vi "test harness_FXP_Linear_controller_observer.vi"(8 "error in (no error)":errorcluster, 11 "TestCase in":refnum<class "FXP_observer_TestCase.lvclass">) -> (0 "error out":errorcluster, 3 "TestCase out":refnum<class "FXP_observer_TestCase.lvclass">)   [LabVIEW 2017, in "FXP_observer_TestCase.lvclass"]
uses:
  FXP_observer_TestCase.lvclass
  <vilib>/rvi/DesktopExecutionNode/Execution/niFpgaDEN_Execute.vi
  <vilib>/rvi/DesktopExecutionNode/DesktopExecutionNode.xnode
panel:
  out "output array":fxp<+/-,51,11>[](array[numeric])
  out "xk_1_2":fxp<+/-,32,8>[](array[numeric])
  out "xerr":fxp<+/-,32,5>[](array[numeric])
  out "error A*x_k_1":errorcluster
  out "Numeric":dbl
  out "del u(k)":fxp<+/-,64,15>
  out "u_k (saturated)":fxp<+/-,32,5>
  out "A*x 2":fxp<+/-,32,7>[](array[numeric])
  out "error (xk_1_1)":errorcluster
  out "error (ydest)":errorcluster
  out "x+y":fxp<+/-,51,11>[](array[numeric])
  out "Az_mat in":fxp<+/-,32,5>[][](array[numeric])
  in  "du_umax":fxp<+/-,18,5>
  in  "xk_1_0":fxp<+/-,32,5>[](array[numeric])=[0.0, 0.0, 0.0, 0.0, 0.0, 0.0, 0.0, 0.0, 0.0, 0.0, 0.0, 0.0, 0.0, 0.0, 0.0, 0.0, 0.0, 0.0, 0.0, 0.0, 0.0, 0.0, 0.0, 0.0, 0.0, 0.0, 0.0, 0.0, 0.0, 0.0, 0.0, 0.0, 0.0, 0.0, 0.0, 0.0, 0.0, 0.0, 0.0, 0.0, 0.0, 0.0, 0.0, 0.0, 0.0, 0.0, 0.0, 0.0, 0.0, 0.0]
  in  "x_u(k)":fxp<+/-,32,8>
  in  "ControlParams_distEst":T1={"umax"=0.0, "NS"=0, "ref_f_VEC"=[0.0, 0.0], "Nu11_22"=[0.0, 0.0], "u0"=[0.0, 0.0]}
  in  "u(k-1)":fxp<+/-,18,5>=0.14501953125
  in  "y(k)":fxp<+/-,18,5>=0.123046875
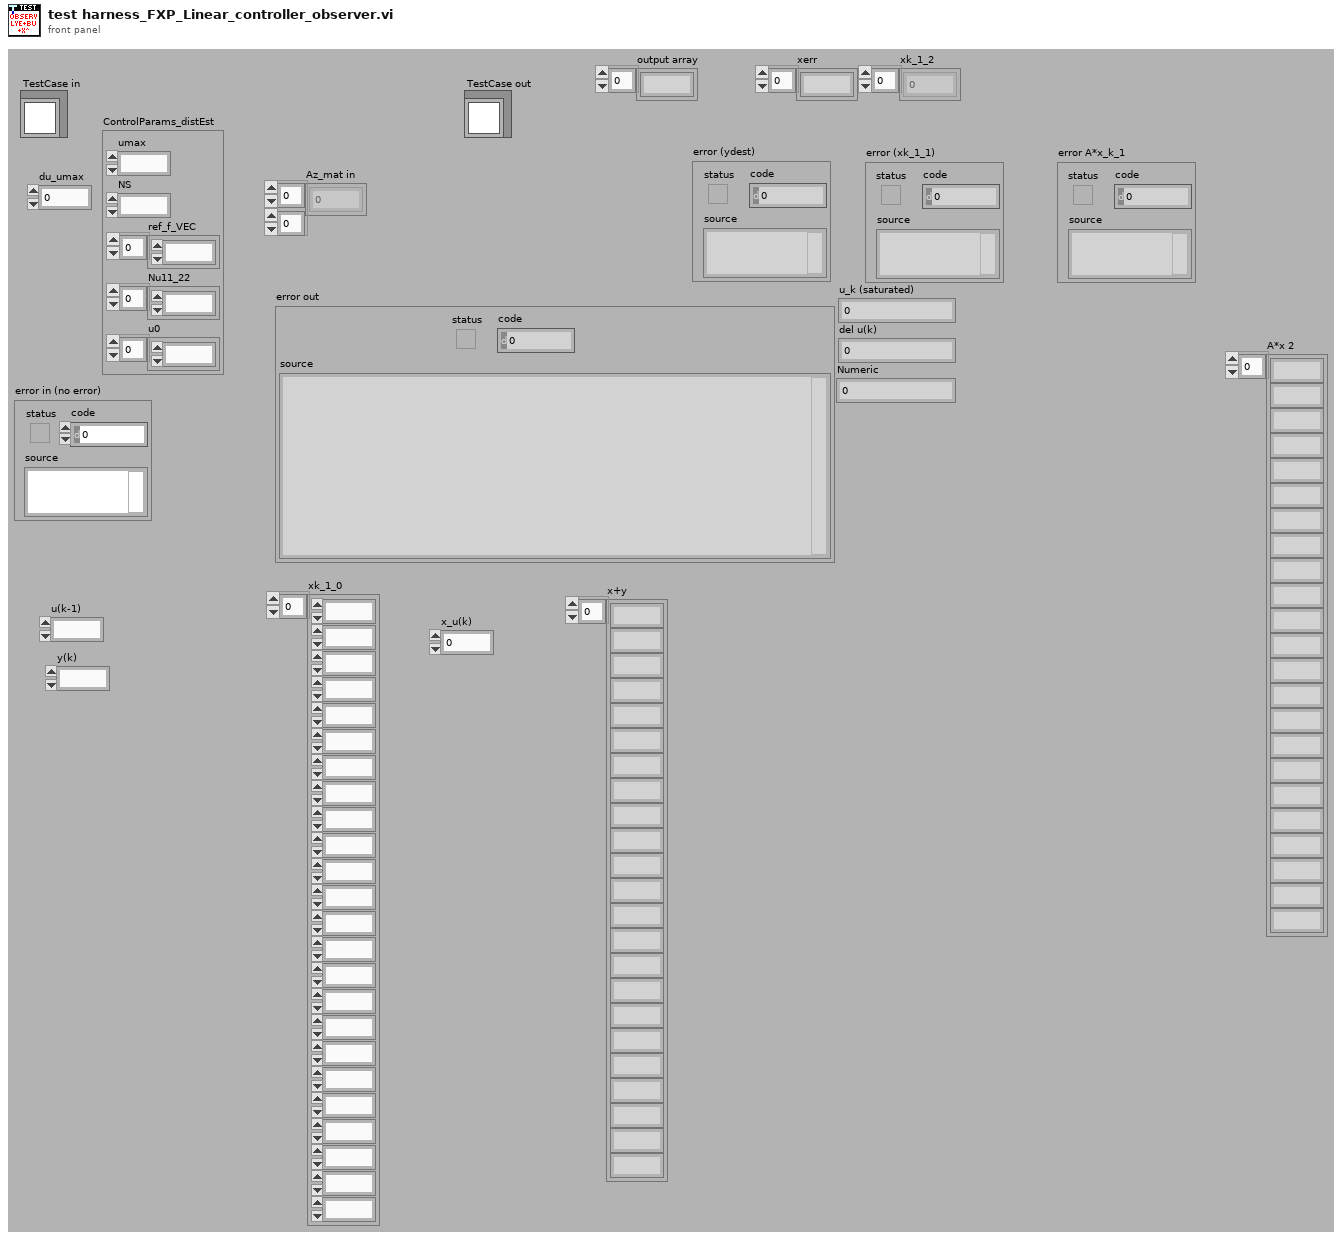
[diagram p1: front panel]
types:
  T1 = cluster{"umax":fxp<+/-,18,5>, "NS":u8, "ref_f_VEC":fxp<+/-,32,5>[], "Nu11_22":fxp<+/-,32,5>[], "u0":fxp<+/-,32,5>[]}
  T2 = cluster{"Bz":fxp<+/-,32,5>[], "Ldist":fxp<+/-,32,5>[], "Kz":fxp<+/-,32,15>[], "Nx":fxp<+/-,32,5>[], "Ax_col":fxp<+/-,32,5>[]}
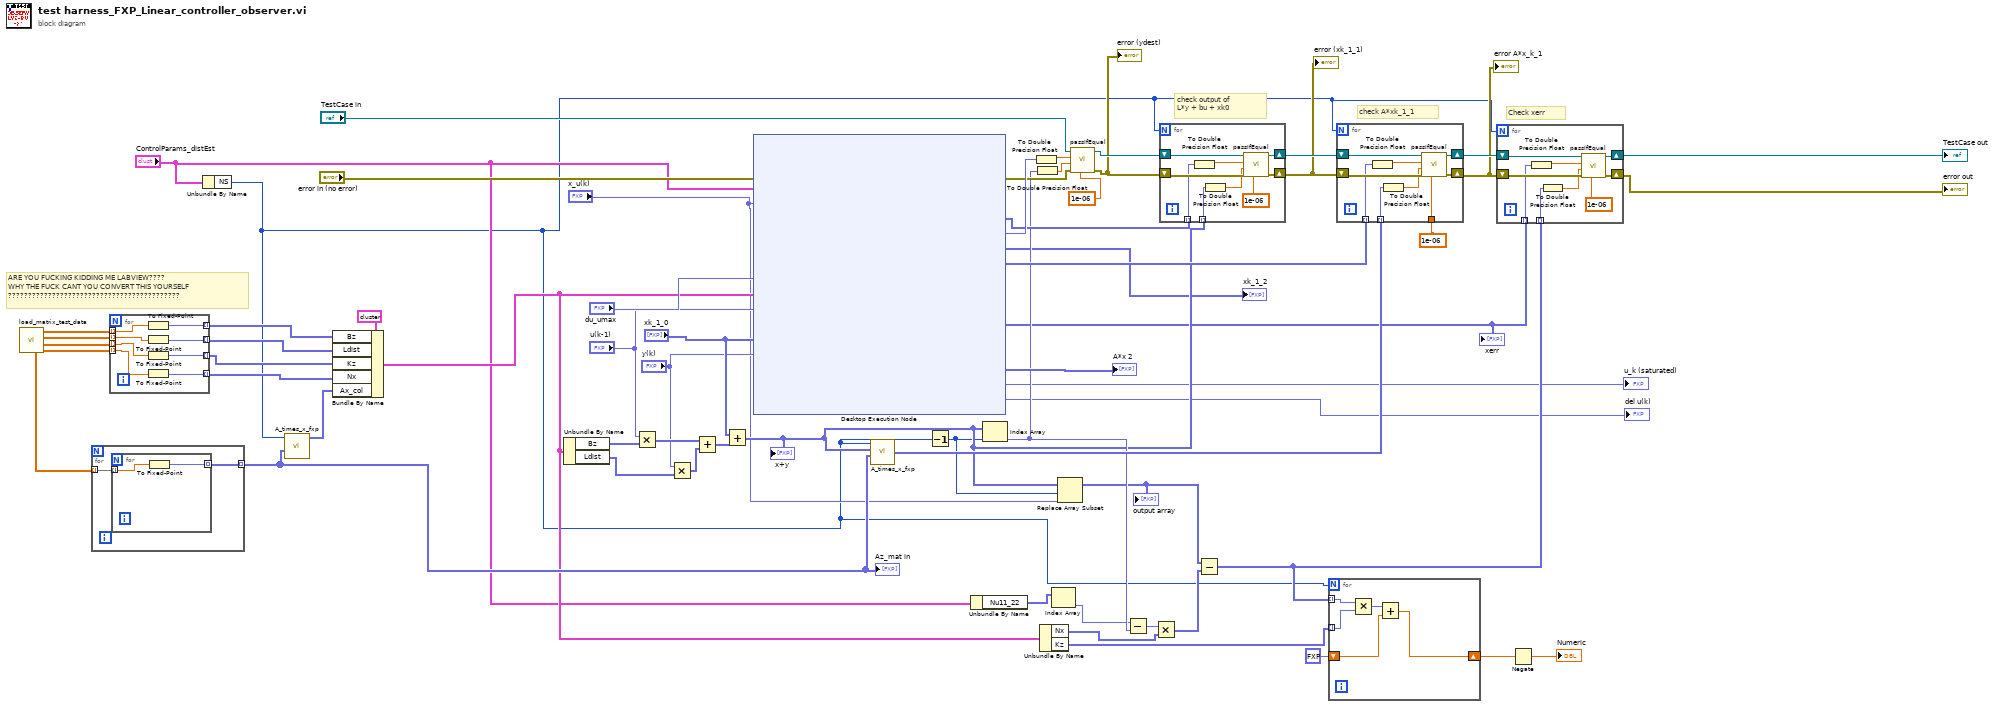
[diagram p0: block diagram]
diagram:
  # "check A*xk_1_1"
  # "check output of \nL*y + bu + xk0"
  # "Check xerr"
  # "ARE YOU FUCKING KIDDING ME LABVIEW????\nWHY THE FUCK CANT YOU CONVERT THIS YOURSELF\n???????????????????????????????????????????"
  n1 = call "load_matrix_test_data.vi"() -> ("Nx"=w57:dbl[], "Kz"=w58:dbl[], "Lz"=w59:dbl[], "Bz"=w60:dbl[], "A_mat"=w56:dbl[][])  [unwired: 5 in, 2 out]
  n2 = for {
    tunnel: [w65] -> w43 mode=indexing
    tunnel: w56 -> [w64] mode=indexing
    n3 = for {
      tunnel: w64 -> [w67] mode=indexing
      tunnel: [w66] -> w65 mode=indexing
      n4 = To Fixed-Point(number=w67) -> (fixed-point=w66:fxp<+/-,32,5>)  [unwired: 1 in]
    }
  }
  "Az_mat in" <- w43
  n5 = for {
    tunnel: w60 -> [w75] mode=indexing
    tunnel: w59 -> [w74] mode=indexing
    tunnel: w58 -> [w73] mode=indexing
    tunnel: w57 -> [w72] mode=indexing
    tunnel: [w71] -> w54 mode=indexing
    tunnel: [w70] -> w53 mode=indexing
    tunnel: [w69] -> w3 mode=indexing
    tunnel: [w68] -> w52 mode=indexing
    n6 = To Fixed-Point(number=w75) -> (fixed-point=w71:fxp<+/-,32,5>)  [unwired: 1 in]
    n7 = To Fixed-Point(number=w74) -> (fixed-point=w70:fxp<+/-,32,5>)  [unwired: 1 in]
    n8 = To Fixed-Point(number=w73) -> (fixed-point=w69:fxp<+/-,32,15>)  [unwired: 1 in]
    n9 = To Fixed-Point(number=w72) -> (fixed-point=w68:fxp<+/-,32,5>)  [unwired: 1 in]
  }
  n10 = Unbundle By Name("ControlParams_distEst") -> ("NS"=w1:u8)
  n11 = call "A_times_x_fxp.vi"("Az_mat in"=w43, "NS"=w1) -> ("Az_vec out"=w51:fxp<+/-,32,5>[])  [unwired: 8 in, 1 out]
  n12 = Bundle By Name(cluster=T2 {"Bz"=[0.0, 0.0, 0.0, 0.0, 0.0, 0.0, 0.0, 0.0, 0.0, 0.0, 0.0, 0.0, 0.0, 0.0, 0.0, 0.0, 0.0, 0.0, 0.0, 0.0, 0.0, 0.0, 0.0, 0.0, 0.0, 0.0, 0.0, 0.0, 0.0, 0.0, 0.0, 0.0, 0.0, 0.0, 0.0, 0.0, 0.0, 0.0, 0.0, 0.0, 0.0, 0.0, 0.0, 0.0, 0.0, 0.0, 0.0, 0.0, 0.0, 0.0], "Ldist"=[0.0, 0.0, 0.0, 0.0, 0.0, 0.0, 0.0, 0.0, 0.0, 0.0, 0.0, 0.0, 0.0, 0.0, 0.0, 0.0, 0.0, 0.0, 0.0, 0.0, 0.0, 0.0, 0.0, 0.0, 0.0, 0.0, 0.0, 0.0, 0.0, 0.0, 0.0, 0.0, 0.0, 0.0, 0.0, 0.0, 0.0, 0.0, 0.0, 0.0, 0.0, 0.0, 0.0, 0.0, 0.0, 0.0, 0.0, 0.0, 0.0, 0.0], "Kz"=[0.0, 0.0, 0.0, 0.0, 0.0, 0.0, 0.0, 0.0, 0.0, 0.0, 0.0, 0.0, 0.0, 0.0, 0.0, 0.0, 0.0, 0.0, 0.0, 0.0, 0.0, 0.0, 0.0, 0.0, 0.0, 0.0, 0.0, 0.0, 0.0, 0.0, 0.0, 0.0, 0.0, 0.0, 0.0, 0.0, 0.0, 0.0, 0.0, 0.0, 0.0, 0.0, 0.0, 0.0, 0.0, 0.0, 0.0, 0.0, 0.0, 0.0], "Nx"=[0.0, 0.0, 0.0, 0.0, 0.0, 0.0, 0.0, 0.0, 0.0, 0.0, 0.0, 0.0, 0.0, 0.0, 0.0, 0.0, 0.0, 0.0, 0.0, 0.0, 0.0, 0.0, 0.0, 0.0, 0.0, 0.0, 0.0, 0.0, 0.0, 0.0, 0.0, 0.0, 0.0, 0.0, 0.0, 0.0, 0.0, 0.0, 0.0, 0.0, 0.0, 0.0, 0.0, 0.0, 0.0, 0.0, 0.0, 0.0, 0.0, 0.0], "Ax_col"=[0.0, 0.0, 0.0, 0.0, 0.0, 0.0, 0.0, 0.0, 0.0, 0.0, 0.0, 0.0, 0.0, 0.0, 0.0, 0.0, 0.0, 0.0, 0.0, 0.0, 0.0, 0.0, 0.0, 0.0, 0.0, 0.0, 0.0, 0.0, 0.0, 0.0, 0.0, 0.0, 0.0, 0.0, 0.0, 0.0, 0.0, 0.0, 0.0, 0.0, 0.0, 0.0, 0.0, 0.0, 0.0, 0.0, 0.0, 0.0, 0.0, 0.0, 0.0, 0.0, 0.0, 0.0, 0.0, 0.0, 0.0, 0.0, 0.0, 0.0, 0.0, 0.0, 0.0, 0.0, 0.0, 0.0, 0.0, 0.0, 0.0, 0.0, 0.0, 0.0, 0.0, 0.0, 0.0, 0.0, 0.0, 0.0, 0.0, 0.0, 0.0, 0.0, 0.0, 0.0, 0.0, 0.0, 0.0, 0.0, 0.0, 0.0, 0.0, 0.0, 0.0, 0.0, 0.0, 0.0, 0.0, 0.0, 0.0, 0.0, 0.0, 0.0, 0.0, 0.0, 0.0, 0.0, 0.0, 0.0, 0.0, 0.0, 0.0, 0.0, 0.0, 0.0, 0.0, 0.0, 0.0, 0.0, 0.0, 0.0, 0.0, 0.0, 0.0, 0.0, 0.0, 0.0, 0.0, 0.0, 0.0, 0.0, 0.0, 0.0, 0.0, 0.0, 0.0, 0.0, 0.0, 0.0, 0.0, 0.0, 0.0, 0.0, 0.0, 0.0, 0.0, 0.0, 0.0, 0.0, 0.0, 0.0, 0.0, 0.0, 0.0, 0.0, 0.0, 0.0, 0.0, 0.0, 0.0, 0.0, 0.0, 0.0, 0.0, 0.0, 0.0, 0.0, 0.0, 0.0, 0.0, 0.0, 0.0, 0.0, 0.0, 0.0, 0.0, 0.0, 0.0, 0.0, 0.0, 0.0, 0.0, 0.0, 0.0, 0.0, 0.0, 0.0, 0.0, 0.0, 0.0, 0.0, 0.0, 0.0, 0.0, 0.0, 0.0, 0.0, 0.0, 0.0, 0.0, 0.0, 0.0, 0.0, 0.0, 0.0, 0.0, 0.0, 0.0, 0.0, 0.0, 0.0, 0.0, 0.0, 0.0, 0.0, 0.0, 0.0, 0.0, 0.0, 0.0, 0.0, 0.0, 0.0, 0.0, 0.0, 0.0, 0.0, 0.0, 0.0, 0.0, 0.0, 0.0, 0.0, 0.0, 0.0, 0.0, 0.0, 0.0, 0.0, 0.0, 0.0, 0.0, 0.0, 0.0, 0.0, 0.0, 0.0, 0.0, 0.0, 0.0, 0.0, 0.0, 0.0, 0.0, 0.0, 0.0, 0.0, 0.0, 0.0, 0.0, 0.0, 0.0, 0.0, 0.0, 0.0, 0.0, 0.0, 0.0, 0.0, 0.0, 0.0, 0.0, 0.0, 0.0, 0.0, 0.0, 0.0, 0.0, 0.0, 0.0, 0.0, 0.0, 0.0, 0.0, 0.0, 0.0, 0.0, 0.0, 0.0, 0.0, 0.0, 0.0, 0.0, 0.0, 0.0, 0.0, 0.0, 0.0, 0.0, 0.0, 0.0, 0.0, 0.0, 0.0, 0.0, 0.0, 0.0, 0.0, 0.0, 0.0, 0.0, 0.0, 0.0, 0.0, 0.0, 0.0, 0.0, 0.0, 0.0, 0.0, 0.0, 0.0, 0.0, 0.0, 0.0, 0.0, 0.0, 0.0, 0.0, 0.0, 0.0, 0.0, 0.0, 0.0, 0.0, 0.0, 0.0, 0.0, 0.0, 0.0, 0.0, 0.0, 0.0, 0.0, 0.0, 0.0, 0.0, 0.0, 0.0, 0.0, 0.0, 0.0, 0.0, 0.0, 0.0, 0.0, 0.0, 0.0, 0.0, 0.0, 0.0, 0.0, 0.0, 0.0, 0.0, 0.0, 0.0, 0.0, 0.0, 0.0, 0.0, 0.0, 0.0, 0.0, 0.0, 0.0, 0.0, 0.0, 0.0, 0.0, 0.0, 0.0, 0.0, 0.0, 0.0, 0.0, 0.0, 0.0, 0.0, 0.0, 0.0, 0.0, 0.0, 0.0, 0.0, 0.0, 0.0, 0.0, 0.0, 0.0, 0.0, 0.0, 0.0, 0.0, 0.0, 0.0, 0.0, 0.0, 0.0, 0.0, 0.0, 0.0, 0.0, 0.0, 0.0, 0.0, 0.0, 0.0, 0.0, 0.0, 0.0, 0.0, 0.0, 0.0, 0.0, 0.0, 0.0, 0.0, 0.0, 0.0, 0.0, 0.0, 0.0, 0.0, 0.0, 0.0, 0.0, 0.0, 0.0, 0.0, 0.0, 0.0, 0.0, 0.0, 0.0, 0.0, 0.0, 0.0, 0.0, 0.0, 0.0, 0.0, 0.0, 0.0, 0.0, 0.0, 0.0, 0.0, 0.0, 0.0, 0.0, 0.0, 0.0, 0.0, 0.0, 0.0, 0.0, 0.0, 0.0, 0.0, 0.0, 0.0, 0.0, 0.0, 0.0, 0.0, 0.0, 0.0, 0.0, 0.0, 0.0, 0.0, 0.0, 0.0, 0.0, 0.0, 0.0, 0.0, 0.0, 0.0, 0.0, 0.0, 0.0, 0.0, 0.0, 0.0, 0.0, 0.0, 0.0, 0.0, 0.0]} ("matrix data"), "Bz"=w54, "Ldist"=w53, "Kz"=w3, "Nx"=w52, "Ax_col"=w51) -> (w28:T2)
  n13 = Unbundle By Name(w28) -> ("Bz"=w49:fxp<+/-,32,5>[], "Ldist"=w47:fxp<+/-,32,5>[])
  n14 = Multiply(x="u(k-1)", y=w49) -> (x*y=w48:fxp<+/-,50,10>[])
  n15 = Multiply(x="y(k)", y=w47) -> (x*y=w46:fxp<+/-,50,10>[])
  n16 = Add(x=w48, y=w46) -> (x+y=w45:fxp<+/-,51,11>[])
  n17 = Add(x="xk_1_0", y=w45) -> (x+y=w20:fxp<+/-,51,11>[])
  "x+y" <- w20
  n18 = xnode "Desktop Execution Node"("Error In"="error in (no error)", "ControlParams_distEst"="ControlParams_distEst", "x_u(k)"="x_u(k)", "du_umax"="du_umax", "matrix data"=w28, "u(k-1)"="u(k-1)", "xk_1_0"="xk_1_0", "y(k-1)"="y(k)") -> ("Error Out"=w33:errorcluster, "xk_1_1"=w35:fxp<+/-,32,5>[], "yd_est"=w38:fxp<+/-,32,5>, "xk_1_2"=→"xk_1_2":fxp<+/-,32,5>[], "xk_1_0 (out)"=w42:fxp<+/-,32,5>[], "xerr"=w13:fxp<+/-,32,5>[], "A*x"=→"A*x 2":fxp<+/-,32,7>[], "u_k (saturated)"=→"u_k (saturated)":fxp<+/-,32,5>, "del u(k)"=→"del u(k)":fxp<+/-,64,15>)
  "xerr" <- w13
  n19 = call "A_times_x_fxp.vi"("Az_mat in"=w43, "x_k"=w20, "NS"=w1) -> ("A*x"=w29:fxp<+/-,64,12>[])  [unwired: 7 in, 1 out]
  n20 = Decrement(x=w1) -> (x-1=w11:u8)
  n21 = Unbundle By Name("ControlParams_distEst") -> ("Nu11_22"=w22:fxp<+/-,32,5>[])
  n22 = Index Array(array=w20, index=w11) -> (element=w26:fxp<+/-,51,11>)
  n23 = To Double Precision Float(number=w38) -> (double precision float=w40:dbl)
  n24 = To Double Precision Float(number=w26) -> (double precision float=w39:dbl)
  n25 = Unbundle By Name(w28) -> ("Nx"=w24:fxp<+/-,32,5>[], "Kz"=w10:fxp<+/-,32,15>[])
  n26 = Index Array(array=w22) -> (element=w21:fxp<+/-,32,5>)  [unwired: 1 in]
  n27 = Replace Array Subset(array=w20, new element="x_u(k)", index=w11) -> (w18:fxp<+/-,51,11>[])
  "output array" <- w18
  n28 = call-dynamic "passIfEqual.vi"("delta (optional)"=1e-06 ("del u_x"), "error in (no error)"=w33, "y"=w39, "x"=w40, "TestCase in"="TestCase in") -> ("error out"=w32:errorcluster, "TestCase out"=w34:refnum<class "FXP_observer_TestCase.lvclass">)  [unwired: 5 in]
  "error (ydest)" <- w32
  n29 = Subtract(x=w21, y=w26) -> (x-y=w25:fxp<+/-,51,11>)
  n30 = Multiply(x=w25, y=w24) -> (x*y=w17:fxp<+/-,64,15>[])
  n31 = for {
    N: w1 -> [_]
    shift-right: [w84] -> w36
    shift-left: w34 -> [w81]
    shift-right: [w83] -> w31
    shift-left: w32 -> [w82]
    tunnel: w20 -> [w78] mode=indexing
    tunnel: w35 -> [w77] mode=indexing
    n32 = To Double Precision Float(number=w77) -> (double precision float=w79:dbl)
    n33 = To Double Precision Float(number=w78) -> (double precision float=w80:dbl)
    n34 = call-dynamic "passIfEqual.vi"("delta (optional)"=1e-06 ("del u_x"), "error in (no error)"=w82, "y"=w80, "x"=w79, "TestCase in"=w81) -> ("error out"=w83:errorcluster, "TestCase out"=w84:refnum<class "FXP_observer_TestCase.lvclass">)  [unwired: 5 in]
  }
  "error (xk_1_1)" <- w31
  n35 = Subtract(x=w18, y=w17) -> (x-y=w12:fxp<+/-,64,16>[])
  n36 = for {
    N: w1 -> [_]
    tunnel: w12 -> [w89] mode=indexing
    tunnel: w10 -> [w88] mode=indexing
    shift-right: [w85] -> w5
    shift-left: fxp<+,32,5> 0.0 -> [w86]
    n37 = Multiply(x=w89, y=w88) -> (x*y=w87:fxp<+/-,64,31>)
    n38 = Add(x=w87, y=w86) -> (x+y=w85:dbl)
  }
  n39 = for {
    N: w1 -> [_]
    shift-right: [w98] -> w16
    shift-left: w36 -> [w95]
    shift-right: [w97] -> w6
    shift-left: w31 -> [w96]
    tunnel: 1e-06 ("del u_x") -> [w92]
    tunnel: w29 -> [w91] mode=indexing
    tunnel: w42 -> [w90] mode=indexing
    n40 = To Double Precision Float(number=w90) -> (double precision float=w93:dbl)
    n41 = To Double Precision Float(number=w91) -> (double precision float=w94:dbl)
    n42 = call-dynamic "passIfEqual.vi"("delta (optional)"=w92, "error in (no error)"=w96, "y"=w94, "x"=w93, "TestCase in"=w95) -> ("error out"=w97:errorcluster, "TestCase out"=w98:refnum<class "FXP_observer_TestCase.lvclass">)  [unwired: 5 in]
  }
  "error A*x_k_1" <- w6
  n43 = for {
    N: w1 -> [_]
    shift-right: [w107] -> w15
    shift-left: w16 -> [w104]
    shift-right: [w106] -> w14
    shift-left: w6 -> [w105]
    tunnel: w12 -> [w101] mode=indexing
    tunnel: w13 -> [w100] mode=indexing
    n44 = To Double Precision Float(number=w100) -> (double precision float=w102:dbl)
    n45 = To Double Precision Float(number=w101) -> (double precision float=w103:dbl)
    n46 = call-dynamic "passIfEqual.vi"("delta (optional)"=1e-06 ("del u_x"), "error in (no error)"=w105, "y"=w103, "x"=w102, "TestCase in"=w104) -> ("error out"=w106:errorcluster, "TestCase out"=w107:refnum<class "FXP_observer_TestCase.lvclass">)  [unwired: 5 in]
  }
  "error out" <- w14
  "TestCase out" <- w15
  n47 = Negate(x=w5) -> (-x=→"Numeric":dbl)
